vi "StringToDataArray.vi"(0 "Data In":string) -> (1 "Good Data":bool, 2 "Data Out":dbl[](array[numeric]))   [LabVIEW 2014]
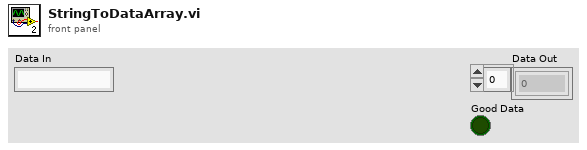
[diagram p1: front panel]
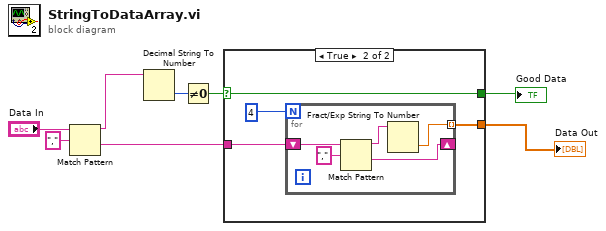
[diagram p0: block diagram]
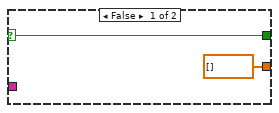
[diagram p2: hidden frame]
diagram:
  n1 = Match Pattern(string="Data In", regular expression=",") -> (before substring=w6:string, after substring=w3:string)  [unwired: 1 in, 2 out]
  n2 = Decimal String To Number(string=w6) -> (number=w5:i32)  [unwired: 2 in, 1 out]
  n3 = Not Equal To 0?(x=w5) -> (x != 0?=w4:bool)
  n4 = case shown="True" w4 {
    selector: w4 -> [w9 w11]
    tunnel: w3 -> [_ w14]
    tunnel: [dbl[] [] w12] -> w2
    tunnel: [w9 w11] -> w1
    frame False {
    }
    frame True {
      n5 = for {
        N: 4 -> [_]
        shift-right: [w17] -> _
        shift-left: w14 -> [w19]
        tunnel: [w15] -> w12 mode=indexing
        n6 = Match Pattern(string=w19, regular expression=",") -> (before substring=w16:string, after substring=w17:string)  [unwired: 1 in, 2 out]
        n7 = Fract/Exp String To Number(string=w16) -> (number=w15:dbl)  [unwired: 3 in, 1 out]
      }
    }
  }
  "Data Out" <- w2
  "Good Data" <- w1
